vi "GetAxilNumber.vi"(8 "error in (no error)":errorcluster, 11 "Stage in":refnum<class "Stage.lvclass">) -> (0 "error out":errorcluster, 2 "Axil Number":dbl, 3 "Stage out":refnum<class "Stage.lvclass">)   [LabVIEW 2020, in "Stage.lvlib" / "Stage.lvclass"]
uses:
  Stage.lvclass
  Stage.lvclass/Stage.ctl
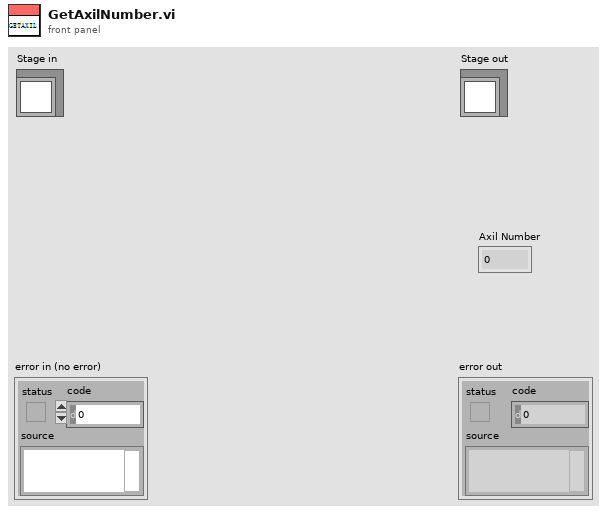
[diagram p1: front panel]
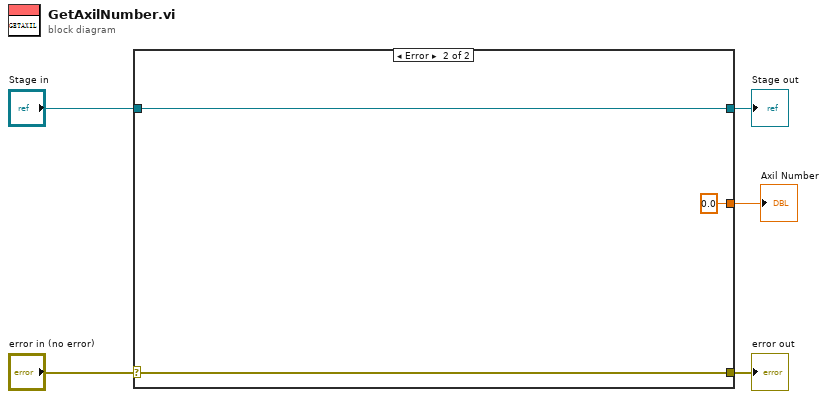
[diagram p0: block diagram]
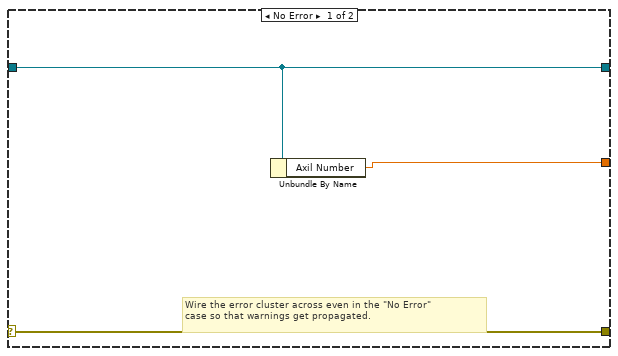
[diagram p2: hidden frame]
diagram:
  n1 = case shown="Error" "error in (no error)" {
    selector: "error in (no error)" -> [w8 w11]
    tunnel: [w8 w11] -> w4
    tunnel: [w7 w10] -> w2
    tunnel: "Stage in" -> [w7 w10]
    tunnel: [w6 0.0 ("Axil Number")] -> w1
    frame No Error {
      # "Wire the error cluster across even in the \"No Error\"\ncase so that warnings get propagated."
      n2 = Unbundle By Name(w7) -> ("Axil Number"=w6:dbl)
    }
    frame Error {
    }
  }
  "error out" <- w4
  "Stage out" <- w2
  "Axil Number" <- w1
